vi "nOfUpTimes.vi"(8 "nOfUpTimes":u16, 9 "signal":bool, 10 "change int":u16, 11 "Tick Count(Ticks)":u16) -> (3 "Boolean":bool)   [LabVIEW 2014]
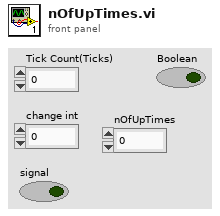
[diagram p1: front panel]
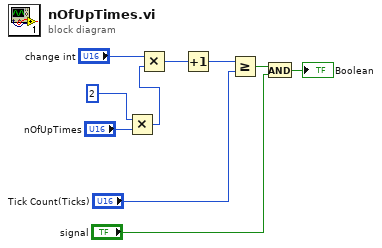
[diagram p0: block diagram]
diagram:
  n1 = Multiply(x=u16 2 ("y"), y="nOfUpTimes") -> (x*y=w2:u16)
  n2 = Multiply(x="change int", y=w2) -> (x*y=w6:u16)
  n3 = Increment(x=w6) -> (x+1=w7:u16)
  n4 = Greater Or Equal?(x=w7, y="Tick Count(Ticks)") -> (x >= y?=w4:bool)
  n5 = And(x=w4, y="signal") -> (x .and. y?=→"Boolean":bool)
